vi "Self Test.vi"(8 "error in (no error)":errorcluster, 11 "NRT8000 in":refnum<class "NRT8000.lvclass">) -> (0 "error out":errorcluster, 2 "Response":string, 3 "NRT8000 out":refnum<class "NRT8000.lvclass">)   [LabVIEW 2018, in "NRT8000.lvlib" / "NRT8000.lvclass"]
uses:
  NRT8000.lvclass
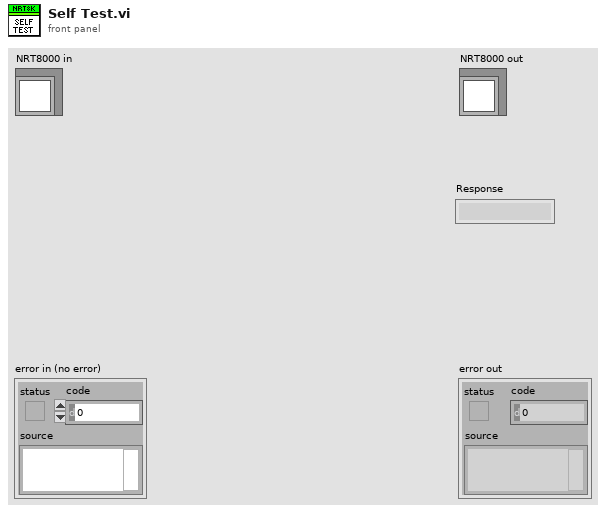
[diagram p1: front panel]
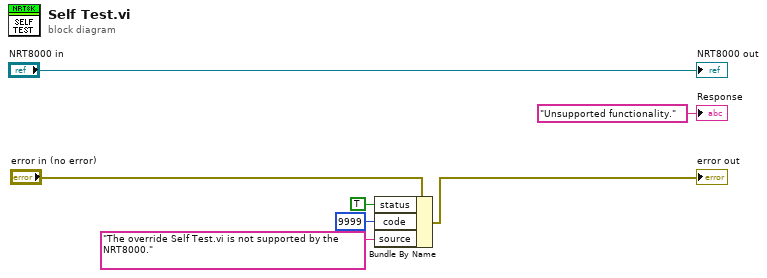
[diagram p0: block diagram]
diagram:
  n1 = Bundle By Name(cluster="error in (no error)", "status"=TRUE, "code"=9999, "source"="The override Self Test.vi is not supported by the NRT8000.") -> (→"error out":errorcluster)
  "NRT8000 out" <- "NRT8000 in"
  "Response" <- "Unsupported functionality." ("Response")
